vi "Process.vi"(8 "error in":errorcluster, 11 "Logger.syslog":refnum<class "Logger.syslog.lvclass">) -> (0 "error out":errorcluster, 3 "Logger.syslog out":refnum<class "Logger.syslog.lvclass">)   [LabVIEW 2019, in "Logger.syslog.lvclass"]
doc: "---------------------------------------------------------------\nJKI State Machine Objects™\nhttp://jki.net/state-machine-objects/\nCopyright (C) 2005-2015, JKI <info@jki.net>\nALL RIGHTS RESERVED"
uses:
  Logger.syslog.lvclass
  C:/Program Files (x86)/National Instruments/LabVIEW 2019/vi.lib/JKI/JKI SMO/SMO/SMO.lvclass
  <vilib>/NI/syslog/_subVIs/TypeDefs/syslog_message_cluster.ctl
  <vilib>/NI/syslog/_subVIs/TypeDefs/syslog_facility_codes.ctl
  <vilib>/NI/syslog/_subVIs/TypeDefs/syslog_severity_codes.ctl
  Typedefs/PrivateEvents--Logger.syslog.syslog message.ctl
  Logger.syslog.lvclass/Logger.syslog.ctl
  <vilib>/JKI/JKI SMO/SMO/SMO.lvclass/SMO.ctl
  <vilib>/JKI/JKI SMO/SMO/Private/ReftoDVR--SMO.vi
  <userlib>/LevyLab/Logger/Logger.lvclass
  <vilib>/JKI/JKI SMO/SMO/SMO.lvclass
panel:
  # "For instructions on how to use the JKI State Machine Objects, examples and video tutorials, visit:\nhttp://jki.net/state-machine-objects/\n\nJKI State Machine Objects™\nhttp://jki.net/state-machine-objects/\nCopyright (C) 2005-2015, JKI <info@jki.net>\nALL RIGHTS RESERVED"
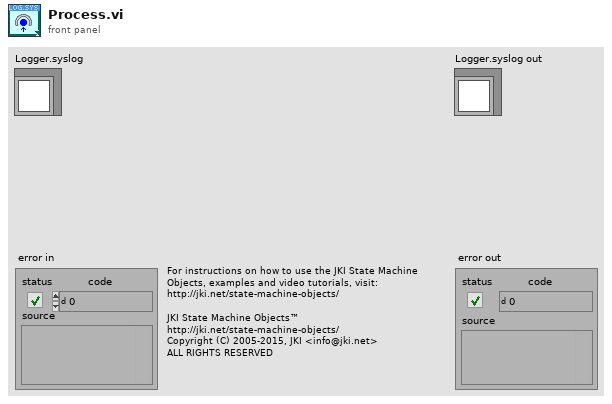
[diagram p1: front panel]
types:
  T1 = enum32{"invalid app kind", "Development System", "Run Time System", "Student Edition", "Embedded LabVIEW", "Evaluation", "Custom"}
  T2 = enum32{"Invalid", "Standard", "Closed", "Hidden", "Minimized", "Maximized"}
  T3 = enum16{"open", "replace", "create", "open or create", "replace or create", "replace or create with confirmation"}
  T4 = typedef "Logger.syslog.lvclass/PrivateEvents--Logger.syslog.syslog message.ctl" = string
  T5 = typedef "syslog_message_cluster.ctl" = cluster{"Facility Code":T6, "Severity Code":T7, "Time Stamp":timestamp, "Hostname":string, "Message Tag":string, "Message Content":string}
  T6 = typedef "syslog_facility_codes.ctl" = enum16{"kernel", "user", "mail", "system daemons", "security/authorization", "syslogd", "line printer", "network news", "uucp", "clock daemon", "security/authorization (alternate)", "FTP daemon", "NTP subsystem", "log audit", "log alert", "clock daemon (alternate)", "local use 0", "local use 1", "local use 2", "local use 3", "local use 4", "local use 5", "local use 6", "local use 7"}
  T7 = typedef "syslog_severity_codes.ctl" = enum16{"emergency", "alert", "critical", "error", "warning", "notice", "info", "debug"}
  T8 = cluster{"Core":cluster{"Current VI Reference":refnum<vi>, "Close Panel on Exit?":bool, "Last Error":cluster{"error":errorcluster, "previous state":string, "remaining states":string}, "Shutdown?":bool}, "SelfRef":refnum<class "Logger.syslog.lvclass">, "collector port (514)":u16, "Syslog Collector Ref":refnum<k16>, "syslog message":T4, "Syslog Message":T5, "path":path}
  T9 = cluster{"Current VI Reference":refnum<vi>, "Close Panel on Exit?":bool, "Last Error":cluster{"error":errorcluster, "previous state":string, "remaining states":string}, "Shutdown?":bool}
  T10 = typedef "SMO.lvclass/Protected Events.ctl" = cluster{"StopProcesses":refnum<user-event>, "AbortProcesses":refnum<user-event>, "Config Changed":refnum<user-event>, "Dependency":refnum<user-event>}
  T11 = typedef "Logger.syslog.lvclass/PrivateEvents--Cluster.ctl" = cluster{"syslog message":refnum<user-event>}
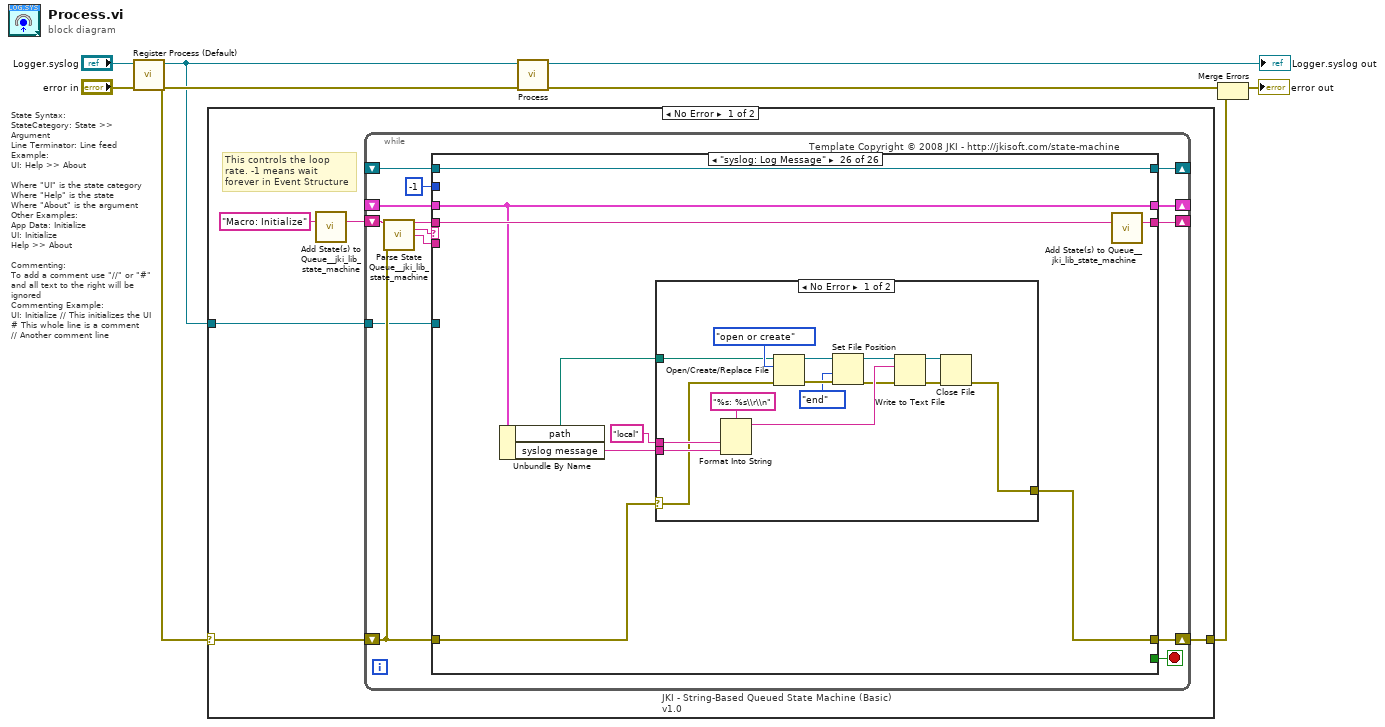
[diagram p0: block diagram]
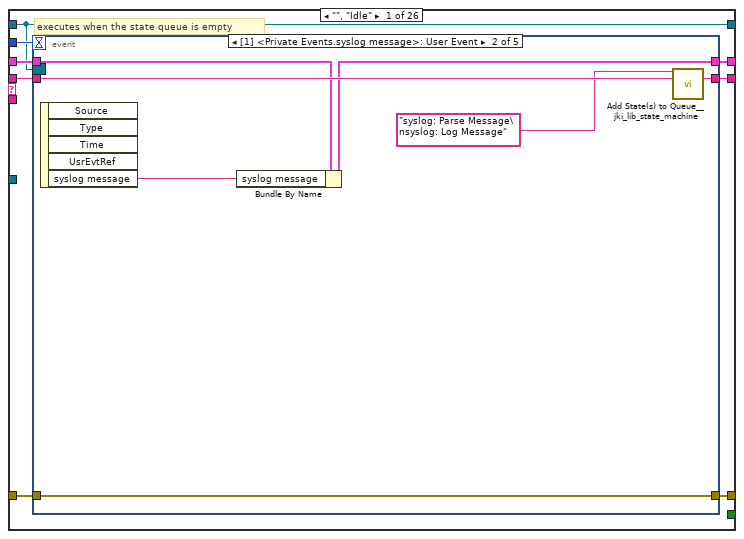
[diagram p2: hidden frame]
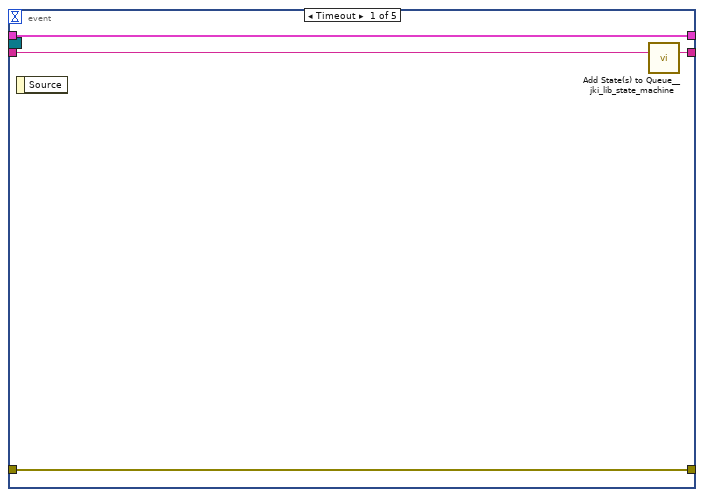
[diagram p3: hidden frame]
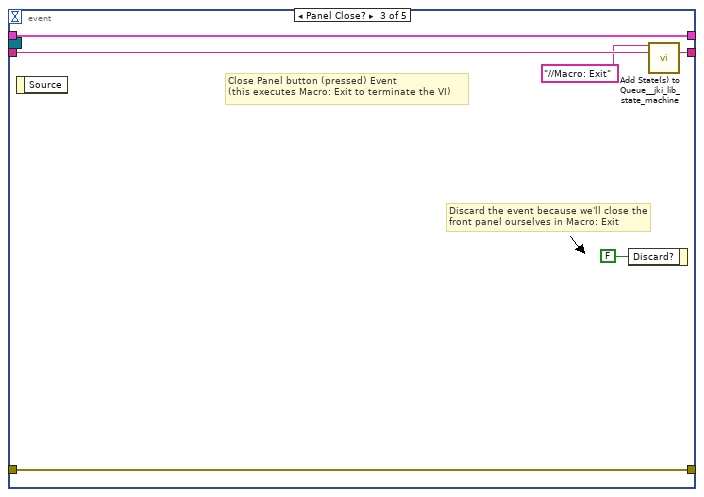
[diagram p4: hidden frame]
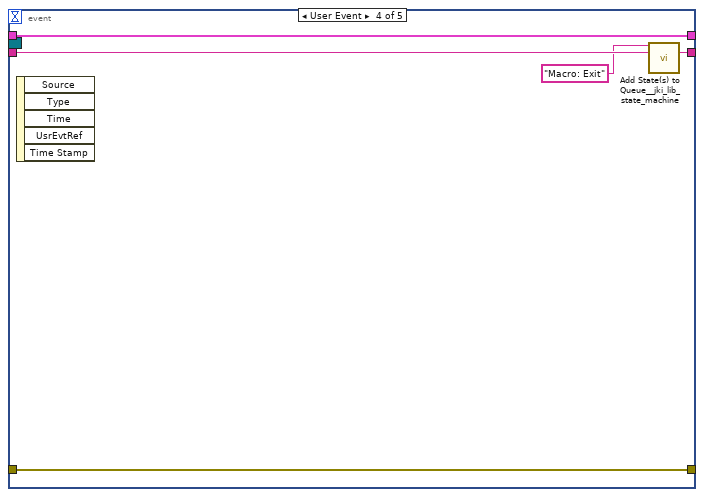
[diagram p5: hidden frame]
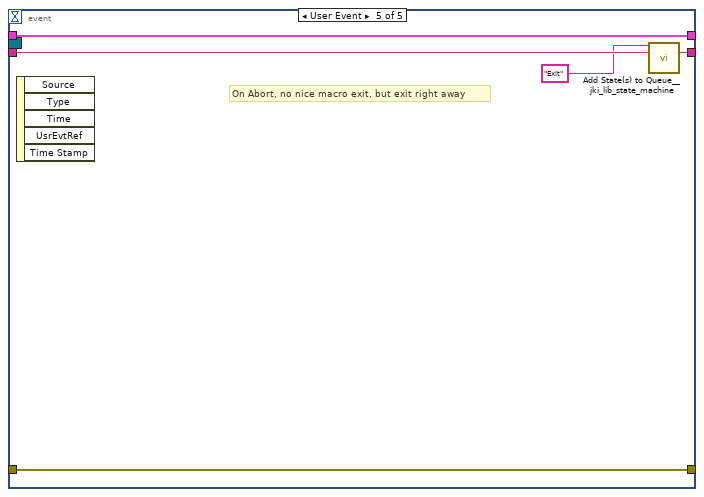
[diagram p6: hidden frame]
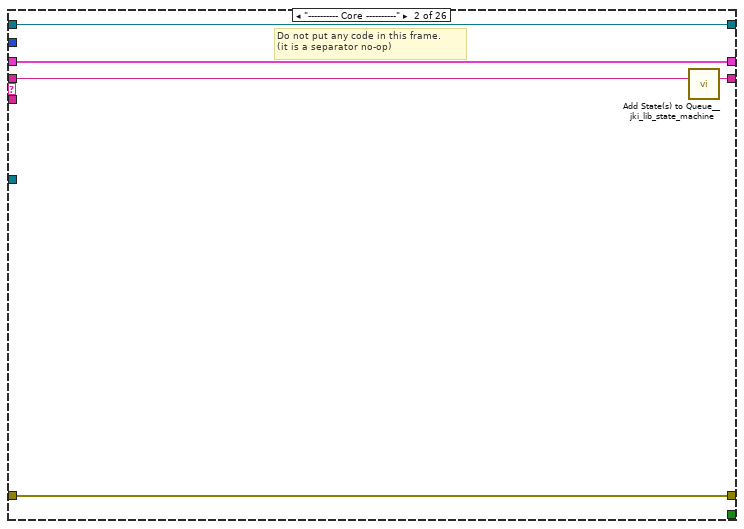
[diagram p7: hidden frame]
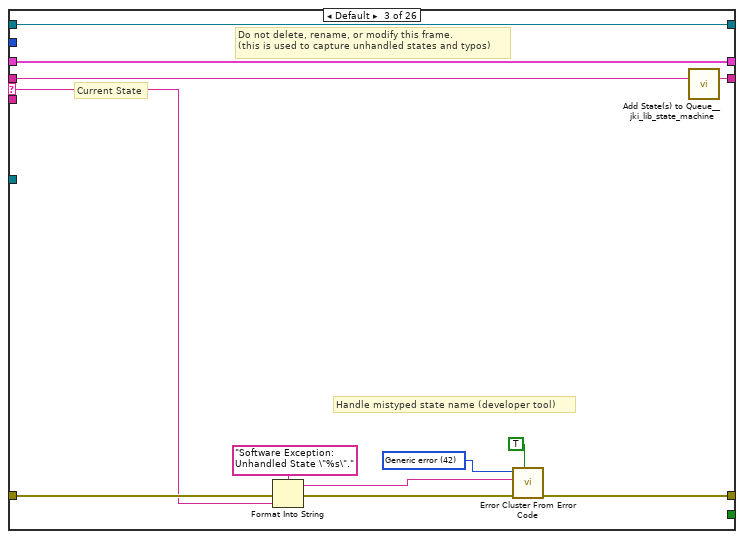
[diagram p8: hidden frame]
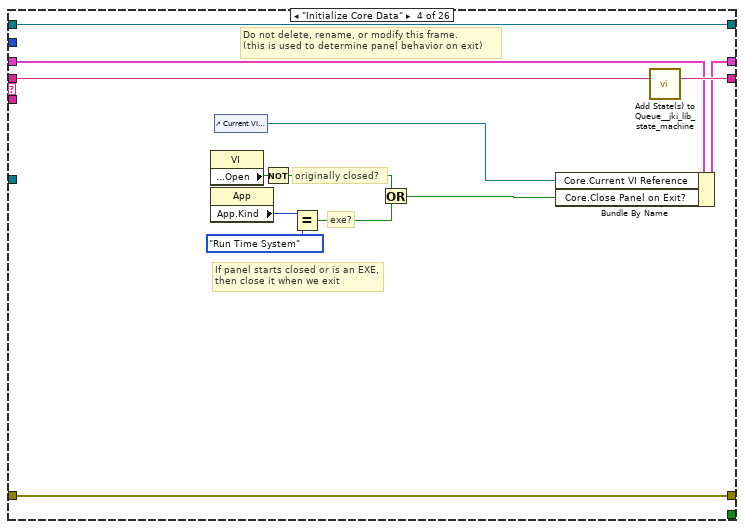
[diagram p9: hidden frame]
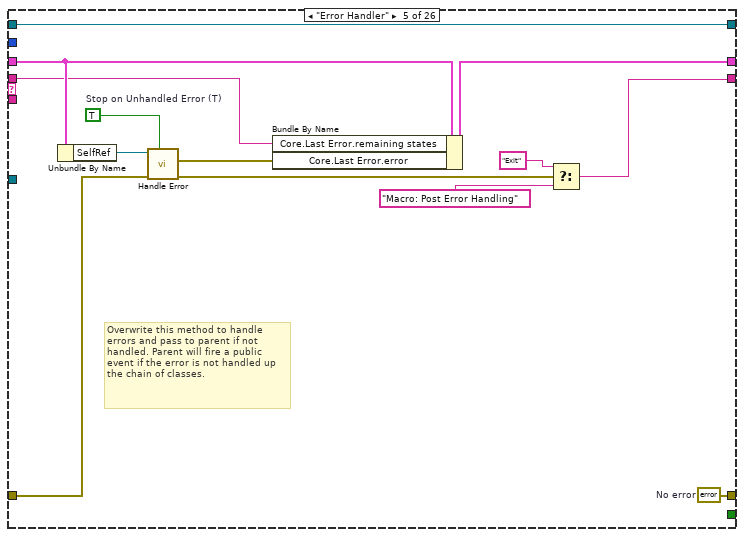
[diagram p10: hidden frame]
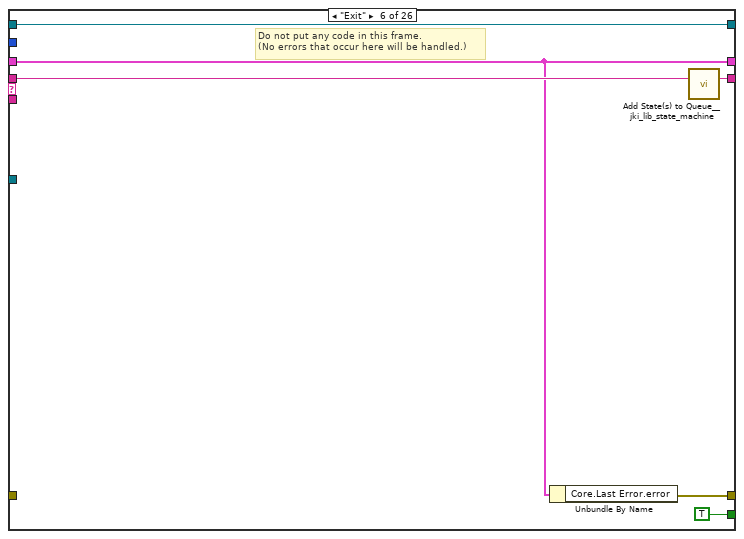
[diagram p11: hidden frame]
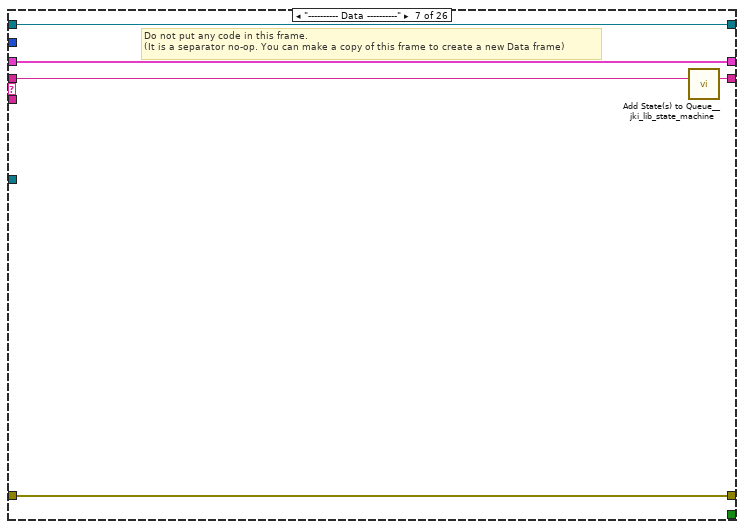
[diagram p12: hidden frame]
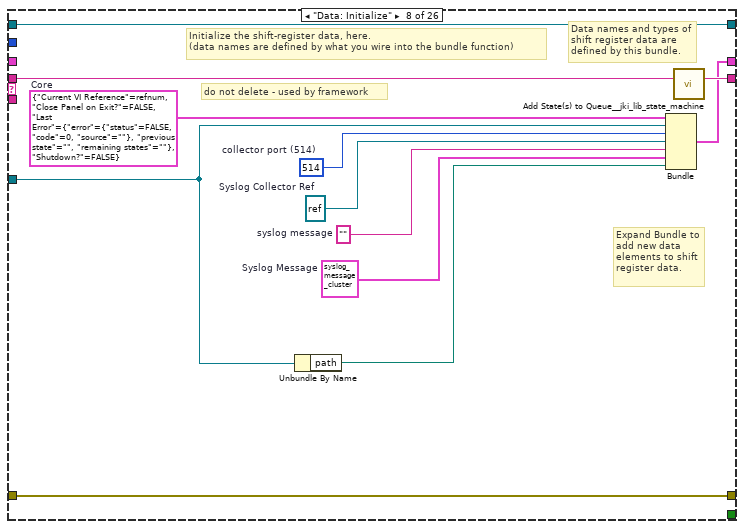
[diagram p13: hidden frame]
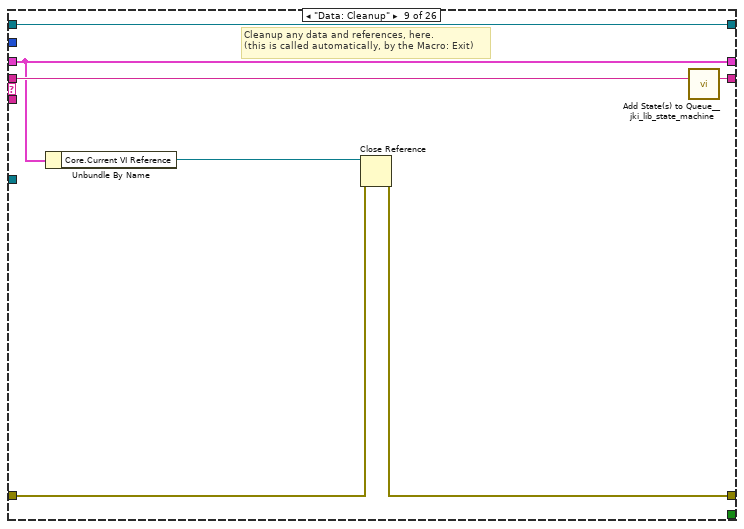
[diagram p14: hidden frame]
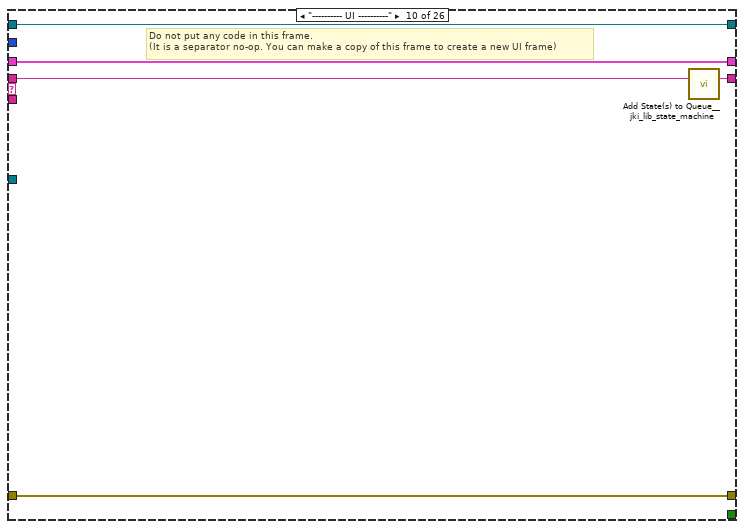
[diagram p15: hidden frame]
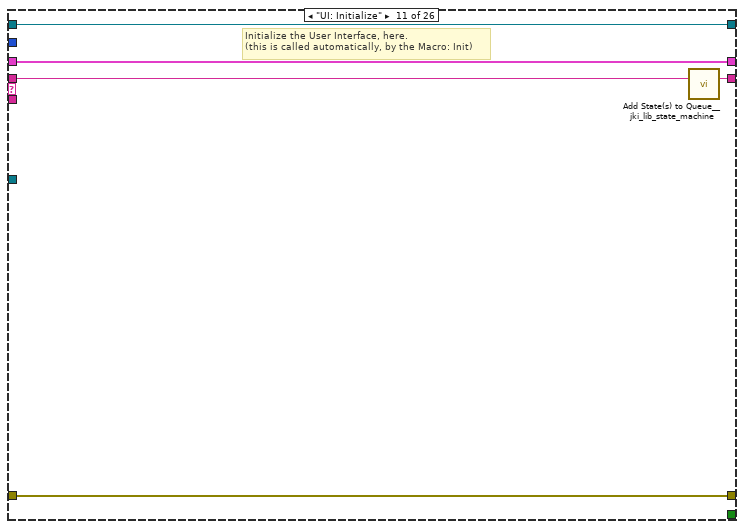
[diagram p16: hidden frame]
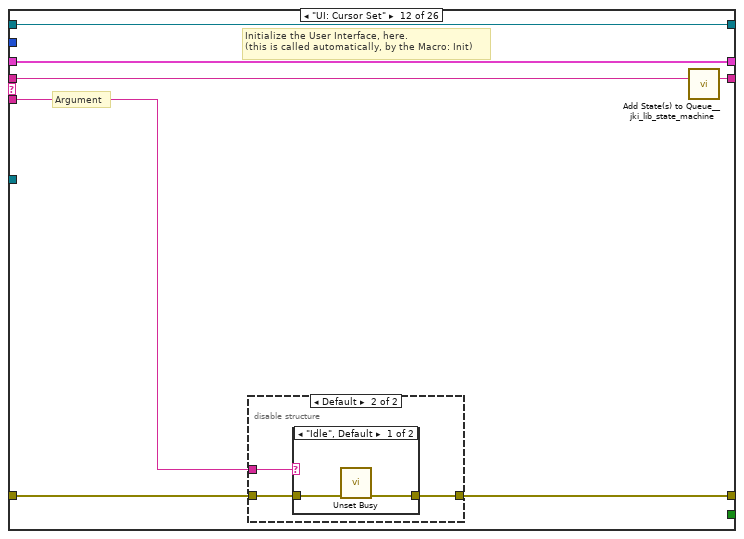
[diagram p17: hidden frame]
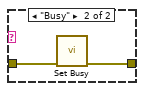
[diagram p19: hidden frame]
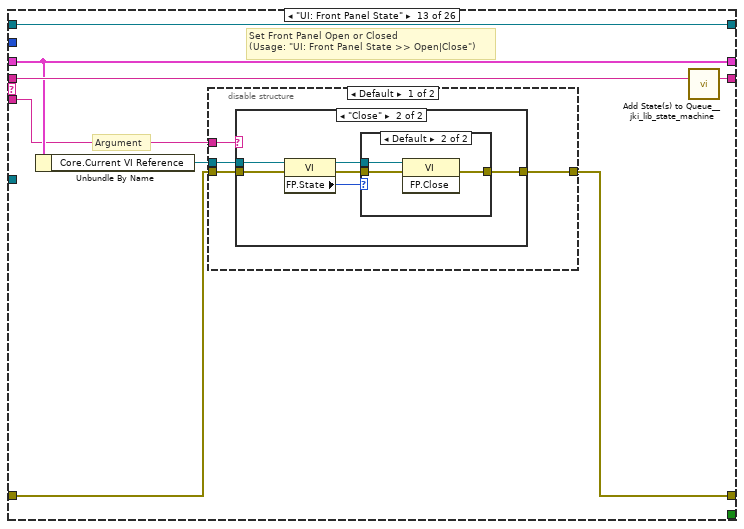
[diagram p20: hidden frame]
diagram:
  # "State Syntax:\nStateCategory: State >> Argument\nLine Terminator: Line feed\nExample:\nUI: Help >> About\n\nWhere \"UI\" is the state category\nWhere \"Help\" is the state\nWhere \"About\" is the argument\nOther Examples:\nApp Data: Initialize\nUI: Initialize\nHelp >> About\n\nCommenting:\nTo add a comment use \"//\" or \"#\" and all text to the right will be ignored\nCommenting Example:\nUI: Initialize // This initializes the UI\n# This whole line is a comment\n// Another comment line"
  n1 = call <vilib>:"Register Process (Default).vi"("error in (no error)"="error in", "SMO"="Logger.syslog") -> ("error out"=w5:errorcluster, "SelfRef"=w4:refnum<class "Logger.syslog.lvclass">)  [unwired: 8 in]
  n2 = case shown="No Error" w5 {
    selector: w5 -> [w10 w332]
    tunnel: w4 -> [w11 _]
    tunnel: [w9 w332] -> w1
    frame No Error {
      # "This controls the loop rate. -1 means wait forever in Event Structure"
      n3 = call <vilib>:"Add State(s) to Queue__jki_lib_state_machine.vi"("State(s) in (\"\")"="Macro: Initialize") -> ("States Out"=w13:string)  [unwired: 14 in]
      n4 = while "JKI - String-Based Queued State Machine (Basic) v1.0" {
        shift-right: [w20] -> _
        shift-left: _ -> [w19]
        shift-right: [w23] -> w9
        shift-left: w10 -> [w17]
        shift-right: [w22] -> _
        shift-left: w13 -> [w24]
        tunnel: w11 -> [w16]
        shift-right: [w15] -> _
        shift-left: _ -> [w14]
        stop <- w21 stop-if-true
        # "Template Copyright © 2008 JKI - http://jkisoft.com/state-machine"
        n5 = call <vilib>:"Parse State Queue__jki_lib_state_machine.vi"("State Queue"=w24, "Error In (no error)"=w17) -> ("Remaining States"=w26:string, "Current State"=w27:string, "Arguments"=w25:string)  [unwired: 11 in]
        n6 = case shown="\"syslog: Log Message\"" w27 {
          selector: w27 -> [_ _ w69 _ _ _ _ _ _ _ _ _ _ _ _ _ _ _ _ _ _ _ _ _ _ _]
          tunnel: w26 -> [w35 w67 w73 w92 w93 w111 w116 w128 w135 w140 w145 w152 w168 w200 w209 w221 w239 w244 w255 w260 w273 w279 w284 w293 w301 w310]
          tunnel: w25 -> [_ _ _ _ _ _ _ _ _ _ _ w146 w162 _ _ _ _ _ _ _ _ _ _ _ _ _]
          tunnel: w19 -> [w33 w64 w71 w83 w101 w107 w113 _ w130 w137 w143 w150 w164 w197 w205 w210 w230 w241 w252 w257 w271 w277 w282 w290 w295 w307]
          tunnel: [w32 w65 w75 w89 w102 w106 w114 w117 w131 w138 w142 w147 w165 w198 w207 w219 w237 w242 w246 w258 w266 w275 w280 w285 w298 w304] -> w23
          tunnel: w17 -> [w31 w65 w74 w89 w103 _ w114 w117 w132 w138 w142 w148 w166 w198 w207 w219 w237 w242 w247 w258 w267 w275 w280 w286 w298 w305]
          tunnel: [w34 w66 w72 w91 w95 w110 w115 w127 w134 w139 w144 w151 w167 w199 w208 w220 w238 w243 w254 w259 w272 w278 w283 w292 w300 w309] -> w22
          tunnel: [_ _ _ _ _ TRUE _ _ _ _ _ _ _ _ _ _ _ _ _ _ _ _ _ _ _ _] -> w21
          tunnel: [w30 w64 w71 w90 w100 w107 w113 w126 w130 w137 w143 w150 w164 w197 w205 w212 w230 w241 w252 w257 w271 w277 w282 w289 w296 w307] -> w20
          tunnel: -1 ("Timeout") -> [w29 _ _ _ _ _ _ _ _ _ _ _ _ _ _ _ _ _ _ _ _ _ _ _ _ _]
          tunnel: w16 -> [_ _ _ _ _ _ _ w118 _ _ _ _ _ _ _ _ _ _ _ _ _ _ _ _ _ _]
          tunnel: [w28 w63 w68 w80 w105 w108 w112 w125 w129 w136 w141 w149 w161 w196 w206 w218 w231 w240 w253 w256 w270 w276 w281 w291 w299 w308] -> w15
          tunnel: w14 -> [w28 w63 w68 w80 w105 w108 w112 w125 w129 w136 w141 w149 w161 w196 w206 w218 w231 w240 w253 w256 _ w276 w281 w291 w299 w308]
          frame "", "Idle" {
            # "executes when the state queue is empty"
            n7 = event shown="[1] <Private Events.syslog message>: User Event" {
              selector: w28 -> [_ _ _ _ _]
              dyn-events: _ -> [_ _ _ _ _]
              timeout: w29 -> [_ _ _ _ _]
              tunnel: w35 -> [w39 w46 w52 w57 w62]
              tunnel: [w38 w45 w51 w56 w61] -> w34
              tunnel: w33 -> [w37 w43 w49 w54 w59]
              tunnel: [w36 w44 w50 w55 w60] -> w32
              tunnel: w31 -> [w36 w44 w50 w55 w60]
              tunnel: [w37 w42 w49 w54 w59] -> w30
              event Timeout {
                n8 = event-data() -> ()  [unwired: 1 in, 1 out]
                n9 = call <vilib>:"Add State(s) to Queue__jki_lib_state_machine.vi"("State(s) in (\"\")"=w39) -> ("States Out"=w38:string)  [unwired: 14 in]
              }
              event User Event {
                n10 = event-data() -> ("syslog message"=w41:T4)  [unwired: 1 in, 4 out]
                n11 = Bundle By Name(cluster=w43, "syslog message"=w41) -> (w42:T8)
                n12 = call <vilib>:"Add State(s) to Queue__jki_lib_state_machine.vi"("State(s) in Front (\"\")"="syslog: Parse Message\nsyslog: Log Message" ("State(s) in Front (\"\")"), "State(s) in (\"\")"=w46) -> ("States Out"=w45:string)  [unwired: 13 in]
              }
              event Panel Close? {
                # "Discard the event because we'll close the front panel ourselves in Macro: Exit"
                # "Close Panel button (pressed) Event\n(this executes Macro: Exit to terminate the VI)"
                n13 = event-data() -> ()  [unwired: 1 in, 1 out]
                n14 = event-data("Discard?"=FALSE) -> ()  [unwired: 1 in, 1 out]
                n15 = call <vilib>:"Add State(s) to Queue__jki_lib_state_machine.vi"("State(s) in Front (\"\")"="//Macro: Exit", "State(s) in (\"\")"=w52) -> ("States Out"=w51:string)  [unwired: 13 in]
              }
              event User Event {
                n16 = event-data() -> ()  [unwired: 1 in, 5 out]
                n17 = call <vilib>:"Add State(s) to Queue__jki_lib_state_machine.vi"("State(s) in Front (\"\")"="Macro: Exit", "State(s) in (\"\")"=w57) -> ("States Out"=w56:string)  [unwired: 13 in]
              }
              event User Event {
                # "On Abort, no nice macro exit, but exit right away"
                n18 = event-data() -> ()  [unwired: 1 in, 5 out]
                n19 = call <vilib>:"Add State(s) to Queue__jki_lib_state_machine.vi"("State(s) in Front (\"\")"="Exit", "State(s) in (\"\")"=w62) -> ("States Out"=w61:string)  [unwired: 13 in]
              }
            }
          }
          frame "---------- Core ----------" {
            # "Do not put any code in this frame.\n(it is a separator no-op)"
            n20 = call <vilib>:"Add State(s) to Queue__jki_lib_state_machine.vi"("State(s) in (\"\")"=w67) -> ("States Out"=w66:string)  [unwired: 14 in]
          }
          frame Default {
            w78 = 42 items=["No error", "Argument error", "Memory is full", "Out of zone", "End of file", "File already open", "Generic file I/O error", "File not found", "File permission error", "Disk is full", "Duplicate path", "Too many files open", "System feature not enabled", "Resource file not found", "Cannot add resource", "Resource not found", "Image not found", "Image memory error", "Pen does not exist", "Config type invalid", "Config token not found", "Config parse error", "Config memory error", "Bad external code format", "Bad external code offset", "External code not present", "Null window", "Destroy window error", "Null menu", "Print aborted", "Bad print record", "Print driver error", "Windows error during printing", "Memory error during printing", "Print dialog error", "Generic print error", "Invalid device refnum", "Device not found", "Device parameter error", "Device unit error", "Cannot open device", "Device call aborted", "Generic error", "Cancelled by user", "Object ID too low", "Object ID too high", "Object not in heap", "Unknown heap", "Unknown object (invalid DefProc)", "Unknown object (DefProc not in table)", "Message out of range", "Invalid (null) method", "Unknown message", "Manager call not supported", "Bad address", "Network operation in progress", "Network operation timed out", "Connection is busy", "Network attribute not supported", "Network error", "Address in use", "System out of memory", "Connection aborted", "Connection refused", "Not connected", "Already connected", "Connection closed", "Initialization error (interapplication manager)", "Bad occurrence", "Wait on unbound occurrence handler", "Occurrence queue overflow", "Datalog type conflict", "Unused", "Unrecognized type (interapplication manager)", "Memory corrupt", "Failed to make temporary DLL", "Old CIN version", "Drag socket not found", "Failed to load drop-object", "Failed to register OLE object", "Failed to release OLE object", "Format specifier type mismatch", "Unknown format specifier", "Too few format specifiers", "Too many format specifiers", "Scan failed", "Newer CIN version", "Error converting to variant", "Runtime menu error", "Password tampered", "Variant attribute not found", "Incompatible variant data type", "Event data is not available", "Event Store is not present", "Occurrence is not found", "Event Queue is not created", "Event info is not available", "Refnum passed is NULL", "Error retrieving Class GUID", "Error retrieving CoClass GUID", "Error retrieving TypeLib GUID.", "Bad built application magic bytes.", "Specific driver is different from the specific driver associated with the Logical Name.", "There is no session opened to the class driver.", "Max Error", "MAX - Error with config objects", "MAX - Error loading configuration", "MAX - Group not supported"]
            # "Current State"
            # "Do not delete, rename, or modify this frame.\n(this is used to capture unhandled states and typos)"
            # "Handle mistyped state name (developer tool)"
            n21 = Format Into String(format string="Software Exception: Unhandled State \"%s\"." ("message"), error in=w74, w69) -> (resulting string=w77:string, error out=w76:errorcluster)  [unwired: 1 in]
            n22 = call <vilib>:"Error Cluster From Error Code.vi"("show call chain? (False)"=TRUE, "error in (no error)"=w76, "error message (\"\")"=w77, "error code (0)"=w78) -> ("error out"=w75:errorcluster)  [unwired: 5 in]
            n23 = call <vilib>:"Add State(s) to Queue__jki_lib_state_machine.vi"("State(s) in (\"\")"=w73) -> ("States Out"=w72:string)  [unwired: 14 in]
          }
          frame "Initialize Core Data" {
            # "Do not delete, rename, or modify this frame.\n(this is used to determine panel behavior on exit)"
            # "originally closed?"
            # "exe?"
            # "If panel starts closed or is an EXE, then close it when we exit"
            n24 = property class="VI"() -> ("Front Panel.Open"=w88:bool)  [unwired: 2 in, 2 out]
            n25 = property class="App"() -> ("App.Kind"=w87:T1)  [unwired: 2 in, 2 out]
            n26 = control-ref of="Current VI Reference"() -> (w81:refnum<vi>)
            n27 = Not(x=w88) -> (.not. x?=w85:bool)
            n28 = Equal?(x=w87, y=T1."Run Time System" ("Application:Kind")) -> (x = y?=w84:bool)
            n29 = Or(x=w85, y=w84) -> (x .or. y?=w82:bool)
            n30 = Bundle By Name(cluster=w83, "Core.Current VI Reference"=w81, "Core.Close Panel on Exit?"=w82) -> (w90:T8)
            n31 = call <vilib>:"Add State(s) to Queue__jki_lib_state_machine.vi"("State(s) in (\"\")"=w92) -> ("States Out"=w91:string)  [unwired: 14 in]
          }
          frame "Error Handler" {
            w96 = TRUE  # Stop on Unhandled Error (T)
            w102 = errorcluster {"status"=FALSE, "code"=0, "source"=""}  # No error
            # "Overwrite this method to handle errors and pass to parent if not handled. Parent will fire a public event if the error is not handled up the chain of classes."
            n32 = Unbundle By Name(w101) -> ("SelfRef"=w104:refnum<class "Logger.syslog.lvclass">)
            n33 = call-dynamic "Handle Error.vi"("Stop on Unhandled Error (T)"=w96, "error in"=w103, "SMO"=w104) -> ("handling error"=w97:errorcluster, "Unhandled error"=w99:errorcluster)  [unwired: 6 in, 1 out]
            n34 = Bundle By Name(cluster=w101, "Core.Last Error.remaining states"=w93, "Core.Last Error.error"=w99) -> (w100:T8)
            n35 = Select(t="Exit", s=w97, f="Macro: Post Error Handling") -> (s? t:f=w95:string)
          }
          frame "Exit" {
            # "Do not put any code in this frame.\n(No errors that occur here will be handled.)"
            n36 = Unbundle By Name(w107) -> ("Core.Last Error.error"=w106:errorcluster)
            n37 = call <vilib>:"Add State(s) to Queue__jki_lib_state_machine.vi"("State(s) in (\"\")"=w111) -> ("States Out"=w110:string)  [unwired: 14 in]
          }
          frame "---------- Data ----------" {
            # "Do not put any code in this frame.\n(It is a separator no-op. You can make a copy of this frame to create a new Data frame)"
            n38 = call <vilib>:"Add State(s) to Queue__jki_lib_state_machine.vi"("State(s) in (\"\")"=w116) -> ("States Out"=w115:string)  [unwired: 14 in]
          }
          frame "Data: Initialize" {
            w121 = T4 ""  # syslog message
            w120 = T5 {"Facility Code"=enum."kernel", "Severity Code"=enum."emergency", "Time Stamp"=timestamp(0 s since 1904-01-01), "Hostname"="", "Message Tag"="", "Message Content"=""}  # Syslog Message
            w122 = refnum<k16> refnum  # Syslog Collector Ref
            w123 = u16 514  # collector port (514)
            w124 = T9 {"Current VI Reference"=refnum, "Close Panel on Exit?"=FALSE, "Last Error"={"error"={"status"=FALSE, "code"=0, "source"=""}, "previous state"="", "remaining states"=""}, "Shutdown?"=FALSE}  # Core
            # "do not delete - used by framework"
            # "Expand Bundle to add new data elements to shift register data."
            # "Data names and types of shift register data are defined by this bundle."
            # "Initialize the shift-register data, here.\n(data names are defined by what you wire into the bundle function)"
            n39 = Unbundle By Name(w118) -> ("path"=w119:path)
            n40 = Bundle("Core"=w124, "SelfRef"=w118, "collector port (514)"=w123, "Syslog Collector Ref"=w122, "syslog message"=w121, "Syslog Message"=w120, "path"=w119) -> (w126:T8)  [unwired: 1 in]
            n41 = call <vilib>:"Add State(s) to Queue__jki_lib_state_machine.vi"("State(s) in (\"\")"=w128) -> ("States Out"=w127:string)  [unwired: 14 in]
          }
          frame "Data: Cleanup" {
            # "Cleanup any data and references, here.\n(this is called automatically, by the Macro: Exit)"
            n42 = Unbundle By Name(w130) -> ("Core.Current VI Reference"=w133:refnum<vi>)
            n43 = Close Reference(reference=w133, error in (no error)=w132) -> (error out=w131:errorcluster)
            n44 = call <vilib>:"Add State(s) to Queue__jki_lib_state_machine.vi"("State(s) in (\"\")"=w135) -> ("States Out"=w134:string)  [unwired: 14 in]
          }
          frame "---------- UI ----------" {
            # "Do not put any code in this frame.\n(It is a separator no-op. You can make a copy of this frame to create a new UI frame)"
            n45 = call <vilib>:"Add State(s) to Queue__jki_lib_state_machine.vi"("State(s) in (\"\")"=w140) -> ("States Out"=w139:string)  [unwired: 14 in]
          }
          frame "UI: Initialize" {
            # "Initialize the User Interface, here.\n(this is called automatically, by the Macro: Init)"
            n46 = call <vilib>:"Add State(s) to Queue__jki_lib_state_machine.vi"("State(s) in (\"\")"=w145) -> ("States Out"=w144:string)  [unwired: 14 in]
          }
          frame "UI: Cursor Set" {
            # "Argument"
            # "Initialize the User Interface, here.\n(this is called automatically, by the Macro: Init)"
            n47 = disable-structure shown="Default" {
              disable-tunnel: w148 -> [w153 w156]
              disable-tunnel: [w153 w155] -> w147
              disable-tunnel: w146 -> [_ w154]
              frame condition #0 {
              }
              frame condition #1 (active) {
                n48 = case shown="\"Idle\", Default" w154 {
                  tunnel: w156 -> [w158 w160]
                  tunnel: [w157 w159] -> w155
                  frame "Idle", Default {
                    n49 = call <vilib>:"Unset Busy.vi"("error in (no error)"=w158) -> ("error out"=w157:errorcluster)  [unwired: 10 in]
                  }
                  frame "Busy" {
                    n50 = call <vilib>:"Set Busy.vi"("error in (no error)"=w160) -> ("error out"=w159:errorcluster)  [unwired: 9 in, 1 out]
                  }
                }
              }
            }
            n51 = call <vilib>:"Add State(s) to Queue__jki_lib_state_machine.vi"("State(s) in (\"\")"=w152) -> ("States Out"=w151:string)  [unwired: 14 in]
          }
          frame "UI: Front Panel State" {
            # "Argument"
            # "Set Front Panel Open or Closed\n(Usage: \"UI: Front Panel State >> Open|Close\")"
            n52 = Unbundle By Name(w164) -> ("Core.Current VI Reference"=w163:refnum<vi>)
            n53 = disable-structure shown="Default" {
              disable-tunnel: w166 -> [w172 w195]
              disable-tunnel: [w171 w195] -> w165
              disable-tunnel: w163 -> [w170 _]
              disable-tunnel: w162 -> [w169 _]
              frame condition #0 (active) {
                n54 = case shown="\"Close\"" w169 {
                  tunnel: w172 -> [w176 w189]
                  tunnel: [w178 w190] -> w171
                  tunnel: w170 -> [w177 w187]
                  frame "Open", Default {
                    n55 = property class="VI"(reference=w177, error in=w176) -> (reference out=w174:refnum<vi>, error out=w175:errorcluster, "FP.State"=w173:T2)
                    n56 = case shown="\"Closed\"" w173 {
                      tunnel: [w181 w184] -> w178
                      tunnel: w175 -> [w180 w184]
                      tunnel: w174 -> [w179 _]
                      frame "Closed" {
                        n57 = invoke class="VI" method="FP.Open"(reference=w179, error in=w180, "Activate"=TRUE, "State"=T2."Standard") -> (error out=w181:errorcluster)  [unwired: 1 in, 4 out]
                      }
                      frame Default {
                      }
                    }
                  }
                  frame "Close" {
                    n58 = property class="VI"(reference=w187, error in=w189) -> (reference out=w186:refnum<vi>, error out=w188:errorcluster, "FP.State"=w185:T2)
                    n59 = case shown="Default" w185 {
                      tunnel: [w191 w194] -> w190
                      tunnel: w188 -> [w191 w193]
                      tunnel: w186 -> [_ w192]
                      frame "Invalid", "Closed" {
                      }
                      frame Default {
                        n60 = invoke class="VI" method="FP.Close"(reference=w192, error in=w193) -> (error out=w194:errorcluster)  [unwired: 1 in, 2 out]
                      }
                    }
                  }
                }
              }
              frame condition #1 {
              }
            }
            n61 = call <vilib>:"Add State(s) to Queue__jki_lib_state_machine.vi"("State(s) in (\"\")"=w168) -> ("States Out"=w167:string)  [unwired: 14 in]
          }
          frame "---------- Macro ----------" {
            # "Do not put any code in this frame.\n(It is a separator no-op. You can make a copy of this frame to create a new Macro frame)"
            n62 = call <vilib>:"Add State(s) to Queue__jki_lib_state_machine.vi"("State(s) in (\"\")"=w200) -> ("States Out"=w199:string)  [unwired: 14 in]
          }
          frame "Macro: Initialize" {
            w203 = "//UI: Initialize\n//UI: Front Panel State >> Open"  # //UI: Initialize //UI: Front Panel State >> Open
            # "Initialization Macro\n(This is called once, when the VI starts)"
            n63 = call <vilib>:"Add State(s) to Queue__jki_lib_state_machine.vi"("State(s) in Front (\"\")"="Data: Initialize\nInitialize Core Data\nEvents: Register", "State(s) in (\"\")"="Process: Sync", "State(s) at Back (\"\")"=w203) -> ("States Out"=w202:string)  [unwired: 12 in]
            n64 = call <vilib>:"Add State(s) to Queue__jki_lib_state_machine.vi"("State(s) in Front (\"\")"=w202, "State(s) in (\"\")"=w209) -> ("States Out"=w208:string)  [unwired: 13 in]
          }
          frame "Macro: Post Error Handling" {
            # "Clear Last Error?"
            n65 = Unbundle By Name(w210) -> ("Core.Last Error.remaining states"=w213:string, "Core.Shutdown?"=w214:bool)
            n66 = Unbundle By Name(w210) -> ("Core.Last Error.error"=w217:errorcluster)
            n67 = case shown="False" FALSE {
              tunnel: w217 -> [w225 _]
              tunnel: [w225 _] -> w216
              frame False {
              }
              frame True {
              }
            }
            n68 = case shown="True" w214 {
              tunnel: w213 -> [w222 w224]
              tunnel: [w222 w223] -> w211
              frame False {
                # "These are the remaining states (at the moment the error occured). States can be altered according to business logic."
                # "NOT SHUTTING DOWN"
              }
              frame True {
                # "Developer can decide to alter the states but should be aware that during the shutdown process, there are certain states that must be run for the SMO to properly shut itself (and this process) down. As such, one can add states to perform additional clean-ups, but should append the remaining state to be executed."
                # "SHUTTING DOWN"
                n69 = call <vilib>:"Add State(s) to Queue__jki_lib_state_machine.vi"("State(s) in (\"\")"=w224) -> ("States Out"=w223:string)  [unwired: 14 in]
              }
            }
            n70 = Bundle By Name(cluster=w210, "Core.Last Error.error"=w216) -> (w212:T8)
            n71 = call <vilib>:"Add State(s) to Queue__jki_lib_state_machine.vi"("State(s) in Front (\"\")"=w211, "State(s) in (\"\")"=w221) -> ("States Out"=w220:string)  [unwired: 13 in]
          }
          frame "Macro: Exit" {
            # "Exit Macro\n(This is called once, when the VI exits)"
            n72 = Unbundle By Name(w230) -> ("Core.Close Panel on Exit?"=w236:bool)
            n73 = Select(t="UI: Front Panel State >> Close", s=w236, f="") -> (s? t:f=w233:string)
            n74 = call <vilib>:"Add State(s) to Queue__jki_lib_state_machine.vi"("State(s) in Front (\"\")"="Data: Cleanup\nEvents: Unregister", "State(s) in (\"\")"="Process: Sync", "State(s) at Back (\"\")"="Exit") -> ("States Out"=w227:string)  [unwired: 12 in]
            n75 = call <vilib>:"Add State(s) to Queue__jki_lib_state_machine.vi"("State(s) in (\"\")"=w233, "State(s) at Back (\"\")"=w227) -> ("States Out"=w232:string)  [unwired: 13 in]
            n76 = call <vilib>:"Add State(s) to Queue__jki_lib_state_machine.vi"("State(s) in Front (\"\")"=w232, "State(s) in (\"\")"=w239) -> ("States Out"=w238:string)  [unwired: 13 in]
          }
          frame "---------- Process ----------" {
            # "Template Separator\n(You can make a copy of, or modify, this frame)"
            n77 = call <vilib>:"Add State(s) to Queue__jki_lib_state_machine.vi"("State(s) in (\"\")"=w244) -> ("States Out"=w243:string)  [unwired: 14 in]
          }
          frame "Process: Sync" {
            n78 = Unbundle By Name(w252) -> ("SelfRef"=w248:refnum<class "Logger.syslog.lvclass">)
            n79 = call <vilib>:"WaitOnProcessSync.vi"("error in (no error)"=w247, "SMO"=w248) -> ("error out"=w246:errorcluster, "Don't run?"=w251:bool)  [unwired: 7 in, 1 out]
            n80 = Select(t="Data: Cleanup\nEvents: Unregister\nExit", s=w251, f="") -> (s? t:f=w245:string)
            n81 = call <vilib>:"Add State(s) to Queue__jki_lib_state_machine.vi"("State(s) in Front (\"\")"=w245, "State(s) in (\"\")"=w255) -> ("States Out"=w254:string)  [unwired: 13 in]
          }
          frame "---------- Events ----------" {
            # "Template Separator\n(You can make a copy of, or modify, this frame)"
            n82 = call <vilib>:"Add State(s) to Queue__jki_lib_state_machine.vi"("State(s) in (\"\")"=w260) -> ("States Out"=w259:string)  [unwired: 14 in]
          }
          frame "Events: Register" {
            # "Expand to add\nmore events"
            n83 = Unbundle By Name(w271) -> ("SelfRef"=w268:refnum<class "Logger.syslog.lvclass">)
            n84 = call <vilib>:"GetProtectedEvents.vi"("SMO"=w268) -> ("error out"=w264:errorcluster, "SMO Protected Events"=w269:T10, "SMO out"=w263:refnum<class "Logger.syslog.lvclass">)  [unwired: 8 in]
            n85 = call "Logger.syslog.GetPrivateEvents.vi"("Logger.syslog"=w263) -> ("error out"=w261:errorcluster, "Private Events"=w262:T11)  [unwired: 8 in, 1 out]
            n86 = register-events(w269, w262) -> (reference out=w270:refnum<event-registration>, error out=w265:errorcluster)  [unwired: 2 in]
            n87 = Merge Errors(w261, w267, w265, w264) -> (w266:errorcluster)
            n88 = call <vilib>:"Add State(s) to Queue__jki_lib_state_machine.vi"("State(s) in (\"\")"=w273) -> ("States Out"=w272:string)  [unwired: 14 in]
          }
          frame "Events: Unregister" {
            n89 = Unregister For Events(event registration refnum=w276, error in=w275) -> (error out=w274:errorcluster)
            n90 = call <vilib>:"Clear Errors.vi"("error in (no error)"=w274) -> ()  [unwired: 5 in, 2 out]
            n91 = call <vilib>:"Add State(s) to Queue__jki_lib_state_machine.vi"("State(s) in (\"\")"=w279) -> ("States Out"=w278:string)  [unwired: 14 in]
          }
          frame "---------- syslog ----------" {
            n92 = call <vilib>:"Add State(s) to Queue__jki_lib_state_machine.vi"("State(s) in (\"\")"=w284) -> ("States Out"=w283:string)  [unwired: 14 in]
          }
          frame "syslog: Start UDP Collector" {
            n93 = Unbundle By Name(w290) -> ("collector port (514)"=w288:u16)
            n94 = call <vilib>:"Syslog Collector Init.vi"("error in (no error)"=w286, "collector port (514)"=w288) -> ("error out"=w285:errorcluster, "Syslog Collector Ref"=w287:refnum<k16>)  [unwired: 8 in]
            n95 = Bundle By Name(cluster=w290, "Syslog Collector Ref"=w287) -> (w289:T8)
            n96 = call <vilib>:"Add State(s) to Queue__jki_lib_state_machine.vi"("State(s) in (\"\")"=w293) -> ("States Out"=w292:string)  [unwired: 14 in]
          }
          frame "syslog: Parse Message" {
            n97 = Unbundle By Name(w295) -> ("syslog message"=w294:T4)
            n98 = call <vilib>:"syslog_Message Parse.vi"("syslog message"=w294) -> ("Syslog Message"=w297:T5)  [unwired: 10 in]
            n99 = Bundle By Name(cluster=w295, "Syslog Message"=w297) -> (w296:T8)
            n100 = call <vilib>:"Add State(s) to Queue__jki_lib_state_machine.vi"("State(s) in (\"\")"=w301) -> ("States Out"=w300:string)  [unwired: 14 in]
          }
          frame "syslog: Log Message" {
            n101 = Unbundle By Name(w307) -> ("path"=w302:path, "syslog message"=w306:T4)
            n102 = case shown="No Error" w305 {
              selector: w305 -> [w312 w326]
              tunnel: w306 -> [w322 _]
              tunnel: [w313 w328] -> w304
              tunnel: "local" ("syslog client address") -> [w323 _]
              tunnel: w302 -> [w311 _]
              frame No Error {
                n103 = Format Into String(format string="%s: %s\\r\\n" ("string"), w323, w322) -> (resulting string=w325:string)  [unwired: 2 in, 1 out]
                n104 = Open/Create/Replace File(file path (use dialog)=w311, error in=w312, operation (0:open)=T3."open or create") -> (refnum out=w318:refnum<file>, error out=w319:errorcluster)  [unwired: 3 in, 1 out]
                n105 = Set File Position(refnum=w318, from (0:start)=enum16{"start", "end", "current"}."end", error in=w319) -> (refnum out=w317:refnum<file>, error out=w320:errorcluster)  [unwired: 1 in]
                n106 = Write to Text File(file (use dialog)=w317, text=w325, error in=w320) -> (refnum out=w315:refnum<file>, error out=w314:errorcluster)  [unwired: 1 in, 1 out]
                n107 = Close File(refnum=w315, error in=w314) -> (error out=w313:errorcluster)  [unwired: 1 out]
              }
              frame Error {
                n108 = Unbundle By Name(w326) -> ("code"=w327:i32)
                n109 = case shown="56" w327 {
                  tunnel: w326 -> [w330 w331]
                  tunnel: [w329 w331] -> w328
                  frame 56 {
                    # "Clear the Timeout error"
                    n110 = call <vilib>:"Clear Errors.vi"("error in (no error)"=w330) -> ("error out"=w329:errorcluster)  [unwired: 5 in, 1 out]
                  }
                  frame Default {
                  }
                }
              }
            }
            n111 = call <vilib>:"Add State(s) to Queue__jki_lib_state_machine.vi"("State(s) in (\"\")"=w310) -> ("States Out"=w309:string)  [unwired: 14 in]
          }
        }
      }
    }
    frame Error {
    }
  }
  n112 = call-parent "Process.vi"("error in"=w5, "SMO"=w4) -> ("error out"=w2:errorcluster, "SMO out"=→"Logger.syslog out":refnum<class "Logger.syslog.lvclass">)  [unwired: 8 in]
  n113 = Merge Errors(w2, w1) -> (→"error out":errorcluster)
